vi "https.put.vi"(6 "specific headers in":cluster{"header":T1, "value":string}[](array[cluster]), 7 "Content Type":string="application/json", 8 "error in":errorcluster, 9 "Body":string, 10 "Path":string, 11 "Nominal Client in":refnum<class "Nominal Client.lvclass">) -> (0 "error out":errorcluster, 2 "Response":string, 3 "Nominal Client out":refnum<class "Nominal Client.lvclass">, 4 "Response Headers":refnum<class "Response Headers.lvclass">)   [LabVIEW 2020, in "Nominal Client.lvclass"]
uses:
  Nominal Client.lvclass
  <vilib>/NI/Advanced HTTP Client/Header--Combo Box.ctl
  <vilib>/addons/_JKI.lib/REST Client/classes/Response Headers/Response Headers.lvclass
  Nominal Client.lvclass/Nominal Client.ctl
  error.vi/859f8e04-e495-489b-b5b4-7ac163f56130.vi
  <vilib>/JDP Science/JSONtext/Get all Object Items.vi
  <vilib>/Utility/error.llb/Error Cluster From Error Code.vi
  <vilib>/JDP Science/JSONtext/JSON text to Variant.vi
  <vilib>/JDP Science/JSONtext/LVClass Serializer/JSONtext LVClass Serializer.lvclass
  <vilib>/addons/_JKI.lib/REST Client/classes/REST Client/REST Client.lvclass
  <vilib>/NI/Advanced HTTP Client/Session.lvclass
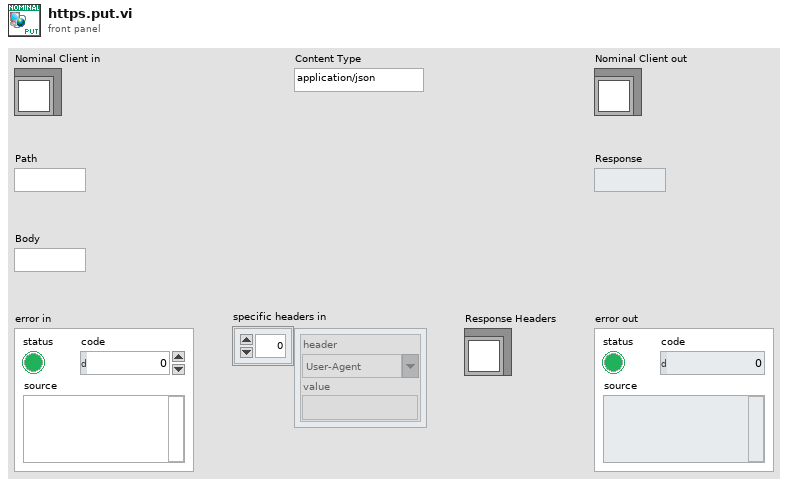
[diagram p1: front panel]
types:
  T1 = typedef "lib_NI_Advanced HTTP Client.lvlib/Session.lvclass/Header--Combo Box.ctl" = string
  T2 = typedef "Nominal Client.lvclass/private_data.ctl" = cluster{"API Token":string, "REST Client":refnum<class "REST Client.lvclass">}
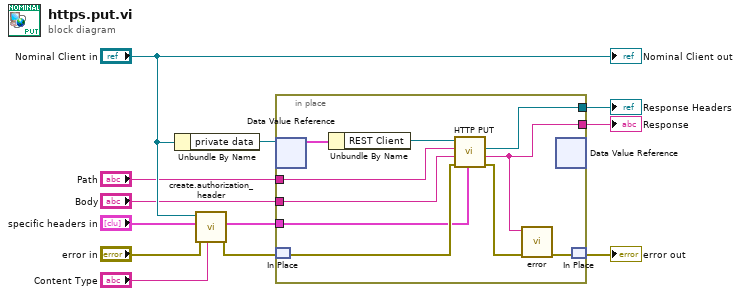
[diagram p0: block diagram]
diagram:
  n1 = Unbundle By Name("Nominal Client in") -> ("private data"=w10:refnum<data-value>)
  n2 = call "create.authorization_header.vi"("Content Type"="Content Type", "error in"="error in", "specific headers in"="specific headers in", "Nominal Client in"="Nominal Client in") -> ("error out"=w5:errorcluster, "specific headers out"=w11:cluster{"header":T1, "value":string}[])  [unwired: 5 in, 1 out]
  n3 = in-place {
    in-place-border: w11 -> [w15]
    in-place-border: [w14] -> w3
    in-place-border: [w19] -> w4
    in-place-border: "Path" -> [w16]
    in-place-border: "Body" -> [w13]
    n4 = in-place-dvr #1(w10) -> (w22:T2)  [unwired: 1 out]
    n5 = in-place-match #2(w5) -> (w18:errorcluster)
    n6 = Unbundle By Name(w22) -> ("REST Client"=w20:refnum<class "REST Client.lvclass">)
    n7 = call-dynamic "HTTP PUT.vi"("request specific headers"=w15, "error in (no error)"=w18, "Request body"=w13, "Path"=w16, "REST Client in"=w20) -> ("error out"=w17:errorcluster, "Response body"=w14:string, "Response Headers"=w19:refnum<class "Response Headers.lvclass">)  [unwired: 1 in, 3 out]
    n8 = call "error.vi"("error in"=w17, "REST Response"=w14) -> ("error out"=w21:errorcluster)  [unwired: 9 in]
    n9 = in-place-dvr #1() -> ()  [unwired: 1 in, 2 out]
    n10 = in-place-match #2(w21) -> (→"error out":errorcluster)
  }
  "Response Headers" <- w4
  "Response" <- w3
  "Nominal Client out" <- "Nominal Client in"
